vi "numericArrayInput.vi"(11 "Array":i32[](array[numeric])) -> (3 "sorted array":dbl[](array[numeric]))   [LabVIEW 2017]
panel:
  in  "Stop Button":bool
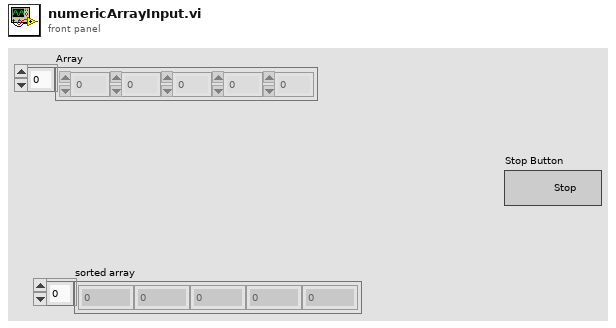
[diagram p1: front panel]
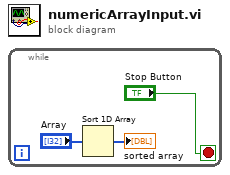
[diagram p0: block diagram]
diagram:
  n1 = while {
    stop <- "Stop Button" stop-if-true
    n2 = Sort 1D Array(array="Array") -> (sorted array=→"sorted array":i32[])
  }
